vi "Write Data to File.vi"(8 "error in (no error)":errorcluster, 10 "File DVR In":T1, 11 "Data in":refnum<class "Data.lvclass">) -> (0 "error out":errorcluster, 2 "File DVR Out":T1, 3 "Data out":refnum<class "Data.lvclass">)   [LabVIEW 2013, in "Base Data Class.lvlib" / "Data.lvclass"]
uses:
  Data.lvclass
  Session APIs/File Access/Base/File Session DVR.ctl
  Session APIs/File Access/Base/File Session.lvclass
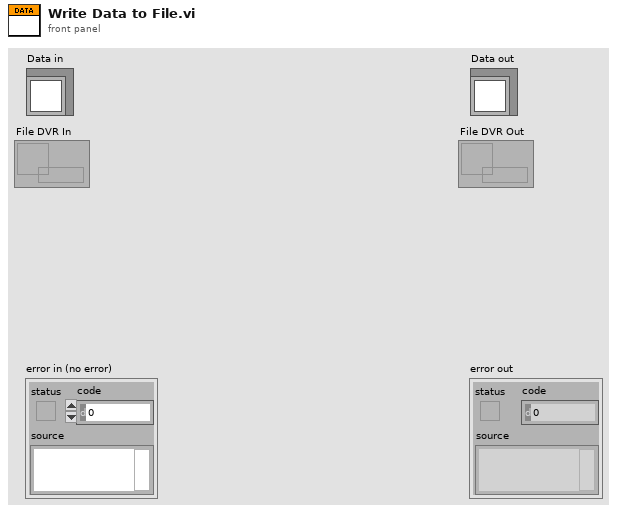
[diagram p1: front panel]
types:
  T1 = typedef "File Session.lvclass/File Session DVR.ctl" = refnum<data-value>
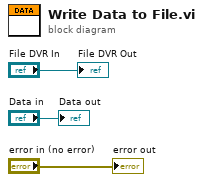
[diagram p0: block diagram]
diagram:
  "error out" <- "error in (no error)"
  "Data out" <- "Data in"
  "File DVR Out" <- "File DVR In"
